vi "Write Time Unit.vi"(8 "error in (no error)":errorcluster, 10 "Time Unit":T1, 11 "Timing Action in":refnum<class "Timing Action.lvclass">) -> (0 "error out":errorcluster, 3 "Timing Action out":refnum<class "Timing Action.lvclass">)   [LabVIEW 2020, in "MacroAssert.lvlib" / "Timing Action.lvclass"]
uses:
  Timing Action.lvclass
  Timing Action.lvclass/Timing Action.ctl
  Time Unit.ctl
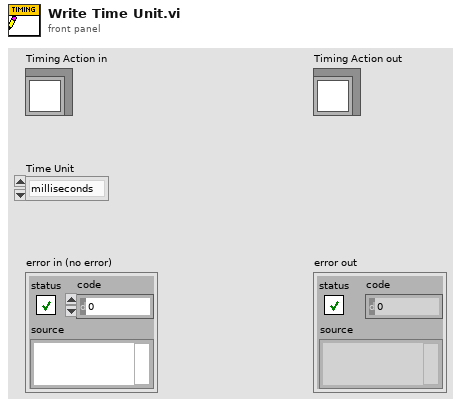
[diagram p1: front panel]
types:
  T1 = typedef "MacroAssert.lvlib/Timing Action.lvclass/Time Unit.ctl" = enum16{"milliseconds", "seconds", "minutes"}
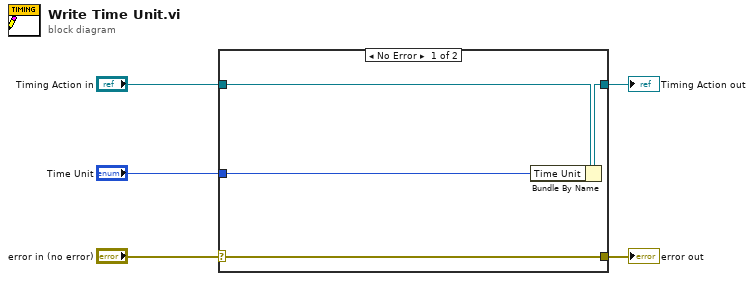
[diagram p0: block diagram]
diagram:
  n1 = case shown="No Error" "error in (no error)" {
    selector: "error in (no error)" -> [w9 w10]
    tunnel: [w9 w10] -> w4
    tunnel: [w7 w11] -> w2
    tunnel: "Timing Action in" -> [w8 w11]
    tunnel: "Time Unit" -> [w6 _]
    frame No Error {
      n2 = Bundle By Name(cluster=w8, "Time Unit"=w6) -> (w7:refnum<class "Timing Action.lvclass">)
    }
    frame Error {
    }
  }
  "error out" <- w4
  "Timing Action out" <- w2
